vi "Enable Buzzer.vi"(8 "error in (no error)":errorcluster, 10 "Buzzer? (T)":bool=TRUE, 11 "VISA resource name":refnum<visa-resource-name>) -> (0 "error out":errorcluster, 3 "VISA resource name out":refnum<visa-resource-name>)   [LabVIEW 2017, in "Siglent SDG 1000 5000 800 Series.lvlib"]
uses:
  <instrlib>/Siglent SDG 1000 5000 800 Series/Siglent SDG 1000 5000 800 Series.lvlib
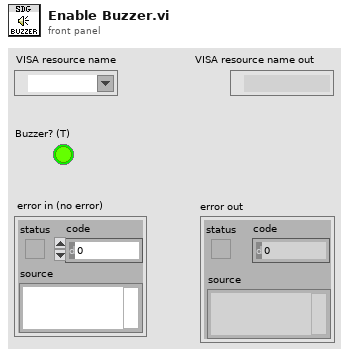
[diagram p1: front panel]
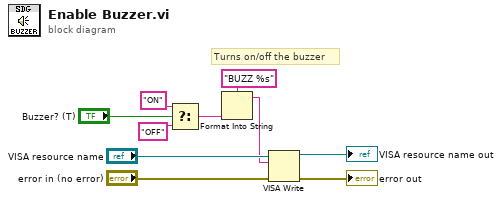
[diagram p0: block diagram]
diagram:
  # "Turns on/off the buzzer"
  n1 = Select(t="ON", s="Buzzer? (T)", f="OFF") -> (s? t:f=w1:string)
  n2 = Format Into String(format string="BUZZ %s", w1) -> (resulting string=w5:string)  [unwired: 2 in, 1 out]
  n3 = VISA Write(VISA resource name="VISA resource name", write buffer=w5, error in (no error)="error in (no error)") -> (VISA resource name out=→"VISA resource name out":refnum<visa-resource-name>, error out=→"error out":errorcluster)  [unwired: 1 out]
